vi "Update Pin Map from XML.vi"(8 "error in":errorcluster, 11 "request data":T2) -> (0 "error out":errorcluster, 3 "response data":T1)   [LabVIEW 2020, in "MeasurementLink Pin Map Client Wrapper.lvlib"]
uses:
  MeasurementLink Pin Map Client Wrapper.lvlib
  Action.ctl
  MeasurementLink Pin Map Client/MeasurementLink Pin Map Client.lvlib
  MeasurementLink Pin Map Client/RPC Messages/ni_measurementlink_pinmap_v1_UpdatePinMapFromXmlRequest.ctl
  MeasurementLink Pin Map Client/RPC Messages/ni_measurementlink_pinmap_v1_PinMap.ctl
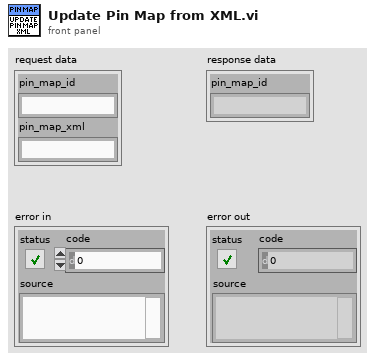
[diagram p1: front panel]
types:
  T1 = typedef "MeasurementLink Pin Map Client.lvlib/ni_measurementlink_pinmap_v1_PinMap.ctl" = cluster{"pin_map_id":string}
  T2 = typedef "MeasurementLink Pin Map Client.lvlib/ni_measurementlink_pinmap_v1_UpdatePinMapFromXmlRequest.ctl" = cluster{"pin_map_id":string, "pin_map_xml":string}
  T3 = typedef "MeasurementLink Pin Map Client Wrapper.lvlib/Action.ctl" = enum16{"Get Client", "Destroy Client"}
  T4 = typedef "grpc-lvsupport-release.lvlib/grpcId.ctl" = u64
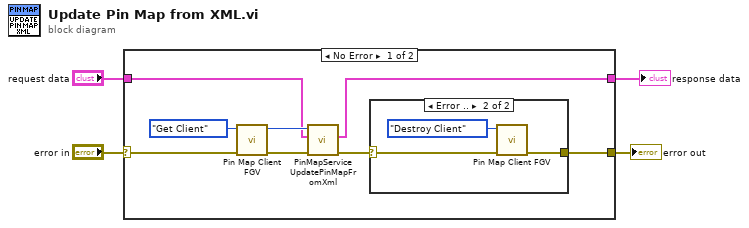
[diagram p0: block diagram]
diagram:
  n1 = case shown="No Error" "error in" {
    selector: "error in" -> [w12 w17]
    tunnel: [w8 w17] -> w3
    tunnel: "request data" -> [w6 _]
    tunnel: [w5 _] -> w1
    frame No Error {
      n2 = call "Pin Map Client FGV.vi"("error in"=w12, "action"=Action."Get Client") -> ("error out"=w11:errorcluster, "grpc client id"=w10:T4)  [unwired: 8 in]
      n3 = call "PinMapService UpdatePinMapFromXml.vi"("error in"=w11, "Request Data"=w6, "gRPC ID"=w10) -> ("error out"=w9:errorcluster, "Response Data"=w5:T1)  [unwired: 6 in, 1 out]
      n4 = case shown="Error .." w9 {
        selector: w9 -> [w13 w16]
        tunnel: [w13 w15] -> w8
        frame No Error {
        }
        frame Error {
          n5 = call "Pin Map Client FGV.vi"("error in"=w16, "action"=Action."Destroy Client") -> ("error out"=w15:errorcluster)  [unwired: 8 in, 1 out]
        }
      }
    }
    frame Error {
    }
  }
  "error out" <- w3
  "response data" <- w1
